vi "traffic_light_v1.vi"() -> ()   [LabVIEW 2019]
panel:
  in  "Stop Button":bool
  out "Rot":bool
  out "Gelb":bool
  out "Grün":bool
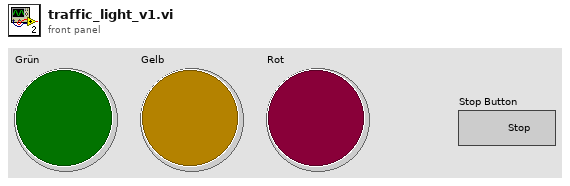
[diagram p1: front panel]
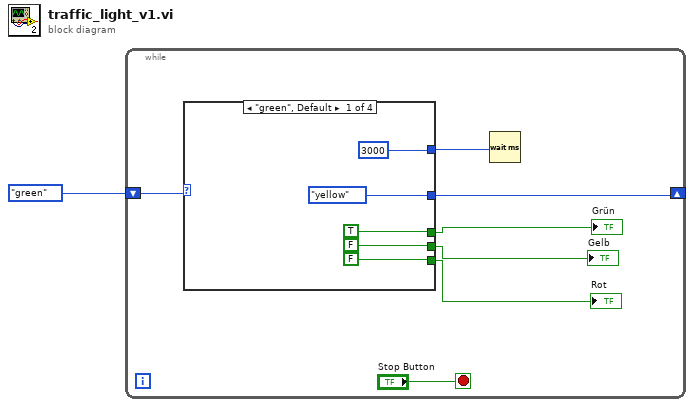
[diagram p0: block diagram]
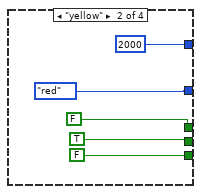
[diagram p2: hidden frame]
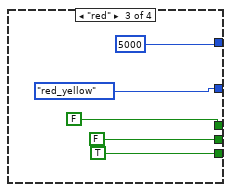
[diagram p3: hidden frame]
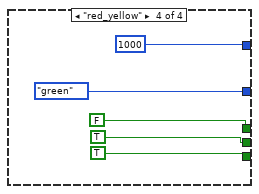
[diagram p4: hidden frame]
diagram:
  n1 = while {
    shift-right: [w5] -> _
    shift-left: enum16{"green", "yellow", "red", "red_yellow"}."green" -> [w7]
    stop <- "Stop Button" stop-if-true
    n2 = case shown="\"green\", Default" w7 {
      tunnel: [3000 2000 5000 1000] -> w6
      tunnel: [FALSE TRUE FALSE TRUE] -> w3
      tunnel: [TRUE FALSE FALSE FALSE] -> w2
      tunnel: [FALSE FALSE TRUE TRUE] -> w4
      tunnel: [enum16{"green", "yellow", "red", "red_yellow"}."yellow" enum16{"green", "yellow", "red", "red_yellow"}."red" enum16{"green", "yellow", "red", "red_yellow"}."red_yellow" enum16{"green", "yellow", "red", "red_yellow"}."green"] -> w5
      frame "green", Default {
      }
      frame "yellow" {
      }
      frame "red" {
      }
      frame "red_yellow" {
      }
    }
    "Grün" <- w2
    "Gelb" <- w3
    "Rot" <- w4
    n3 = Wait (ms)(milliseconds to wait=w6) -> ()  [unwired: 1 out]
  }
